vi "Measurement Selection Icons.vi"() -> (2 "Checked":i32=38, 3 "Unchecked":i32=37)   [LabVIEW 2021, in "MeasurementClient Editor.lvlib"]
uses:
  MeasurementClient Editor.lvlib
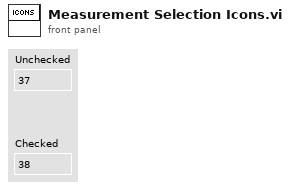
[diagram p1: front panel]
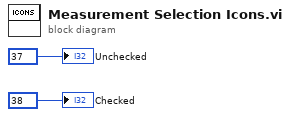
[diagram p0: block diagram]
diagram:
  "Unchecked" <- 37
  "Checked" <- 38
